vi "test_vim_add.vi"() -> ()   [LabVIEW 2018]
uses:
  8d7c883f-3c7e-4aec-8057-698d96ba9072.vi
panel:
  out "Numeric":i32
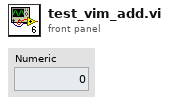
[diagram p1: front panel]
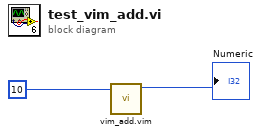
[diagram p0: block diagram]
diagram:
  n1 = call "vim_add.vim"("Variant"=10) -> ("Variant 2"=→"Numeric":i32)  [unwired: 10 in]
